vi "Responder.vi"(8 "error in":errorcluster {"code" format="Error %.0f"}) -> (0 "error out":errorcluster)   [LabVIEW 2024]
uses:
  NATS Subscription/NATS Subscription.lvclass/NATS Subscription.ctl
  NATS Client/NATS Client.lvclass/NATS Client.ctl
  <vilib>/NATS/NATS Core/VIs/NATS CLOSE.vi
  NATS Client/get async stop notifier.vi
  NATS Client/Get Connection DVR.vi
  NATS Client/get subscriptions queue.vi
  NATS Client/Get subscription map.vi
  NATS Client/Get error queue.vi
  NATS Subscription/NATS Subscription.lvclass
  NATS Client/NATS Client.lvclass
panel:
  out "Responding":bool
  # "Instructions:\n\nRun this VI then run Requester.vi.\n\nThis VI will repond to requests."
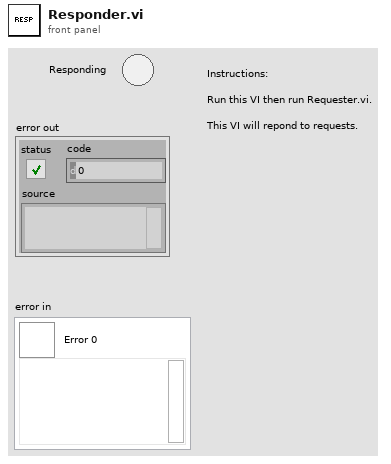
[diagram p1: front panel]
types:
  T1 = typedef "NATS Core.lvlib/nats message.ctl" = cluster{"subject":string, "payload":string, "sub id":string, "reply-to":string, "headers":string, "type":T2, "received":timestamp}
  T2 = typedef "NATS Core.lvlib/msg type.ctl" = enum16{"Undefined", "MSG", "HMSG", "+OK", "PING", "PONG", "-ERR", "INFO"}
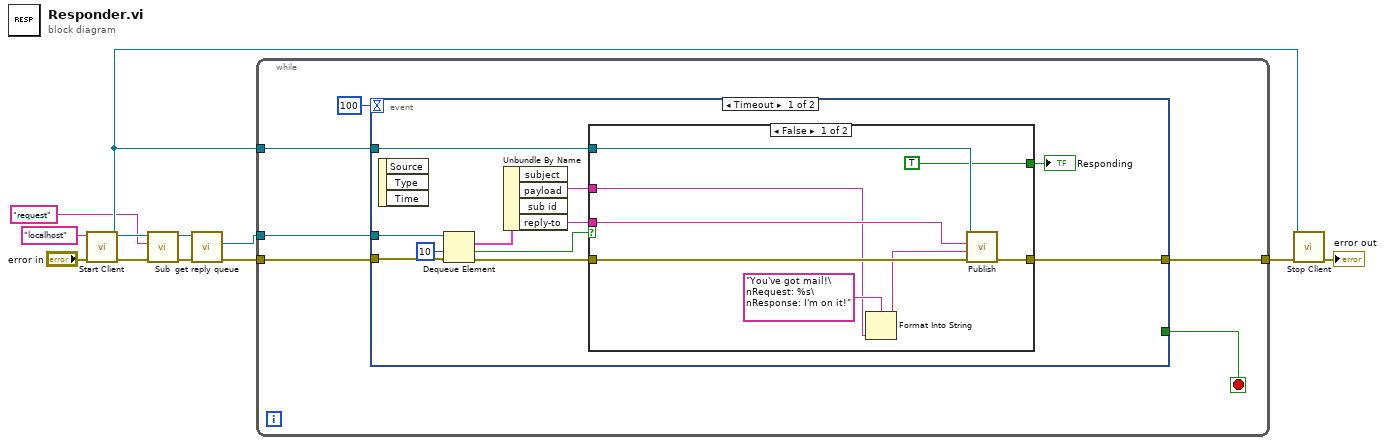
[diagram p0: block diagram]
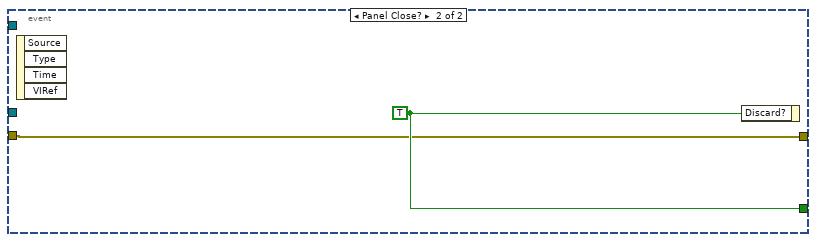
[diagram p3: hidden frame]
diagram:
  n1 = call "Start Client.vi"("error in"="error in", "address"="localhost") -> ("error out"=w7:errorcluster, "NATS Client out"=w8:refnum<class "NATS Client.lvclass">)  [unwired: 8 in]
  n2 = call "Sub.vi"("error in"=w7, "subject"="request" ("Request Subject"), "NATS Client"=w8) -> ("error out"=w2:errorcluster, "NATS Subscription"=w6:refnum<class "NATS Subscription.lvclass">)  [unwired: 7 in]
  n3 = call "get reply queue.vi"("error in"=w2, "NATS Subscription in"=w6) -> ("error out"=w5:errorcluster, "reply queue"=w4:refnum<queue>)  [unwired: 7 in, 1 out]
  n4 = while {
    tunnel: w8 -> [w17]
    tunnel: [w16] -> w10
    tunnel: w5 -> [w14]
    tunnel: w4 -> [w13]
    stop <- w12 stop-if-true
    n5 = event shown="[0] Timeout" {
      selector: _ -> [_ _]
      dyn-events: _ -> [_ _]
      timeout: 100 -> [_ _]
      tunnel: w14 -> [w28 w38]
      tunnel: w17 -> [w27 _]
      tunnel: [w22 w38] -> w16
      tunnel: w13 -> [w21 _]
      tunnel: [_ w39] -> w12
      event Timeout {
        n6 = event-data() -> ()  [unwired: 1 in, 3 out]
        n7 = Dequeue Element(queue=w21, timeout in ms (-1)=10, error in (no error)=w28) -> (element=w25:T1, timed out?=w19:bool, error out=w26:errorcluster)  [unwired: 1 out]
        n8 = Unbundle By Name(w25) -> ("payload"=w23:string, "reply-to"=w24:string)  [unwired: 2 out]
        n9 = case shown="False" w19 {
          tunnel: w27 -> [w36 _]
          tunnel: w26 -> [w35 w37]
          tunnel: w24 -> [w34 _]
          tunnel: w23 -> [w32 _]
          tunnel: [w30 w37] -> w22
          tunnel: [TRUE ("Responding") _] -> w18
          frame False {
            n10 = Format Into String(format string="You've got mail!\nRequest: %s\nResponse: I'm on it!", w32) -> (resulting string=w31:string)  [unwired: 2 in, 1 out]
            n11 = call "Publish.vi"("error in"=w35, "payload"=w31, "subject"=w34, "NATS Client.lvlib:NATS Client.lvclass"=w36) -> ("error out"=w30:errorcluster)  [unwired: 7 in]
          }
          frame True {
          }
        }
        "Responding" <- w18
      }
      event Panel Close? {
        w39 = TRUE ("Discard?")
        n12 = event-data() -> ()  [unwired: 1 in, 4 out]
        n13 = event-data("Discard?"=w39) -> ()  [unwired: 1 in, 1 out]
      }
    }
  }
  n14 = call "Stop Client.vi"("error in"=w10, "NATS Client"=w8) -> ("error out"=→"error out":errorcluster)  [unwired: 9 in]
